vi "GetViableCoordinate.vi"(2 "Target Region [0-3]":i32, 3 "Actual Target Strip [0-1279]":i32) -> (0 "Offset":i32, 1 "Move Probecard to Strip #":i32)   [LabVIEW 2019]
uses:
  ProbePlanParams.vi
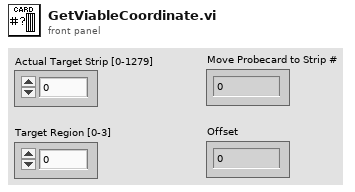
[diagram p1: front panel]
types:
  T1 = cluster{"Strip Number OUT":i32, "X0":i32, "Y0":i32, "X1":i32, "Y1":i32, "Xref":dbl, "Yref":dbl, "ProbePlan type":u32, "Inner pads offset":ext, "Outer pads offset":ext, "l_inner":ext, "l_outer":ext, "strip numbering":u16, "Device Orientation":ext, "Stagger offset":i32, "Yoffset":dbl, "Strip pitch":dbl, "Fiducail separation":dbl, "Radius":ext, "Relative strip angles":dbl, "Probeplan description":string, "ProbePlan array":cluster{"Region":string, "ProbePoints":cluster{"X":dbl, "Y":dbl, "Label":string, "CardViable?":bool}[]}[], "Test ProbePoints":cluster{"Regions Enabled":bool[], "From index":u32[], "To index":u32[]}}
  T2 = cluster{"Region":string, "ProbePoints":cluster{"X":dbl, "Y":dbl, "Label":string, "CardViable?":bool}[]}[]
  T3 = cluster{"Region":string, "ProbePoints":cluster{"X":dbl, "Y":dbl, "Label":string, "CardViable?":bool}[]}
  T4 = cluster{"X":dbl, "Y":dbl, "Label":string, "CardViable?":bool}[]
  T5 = cluster{"X":dbl, "Y":dbl, "Label":string, "CardViable?":bool}
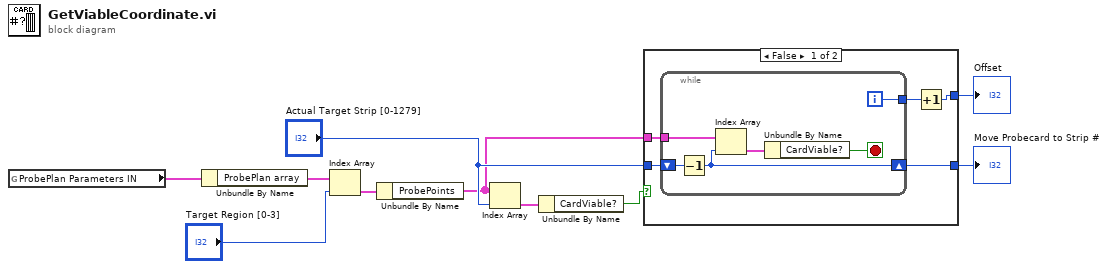
[diagram p0: block diagram]
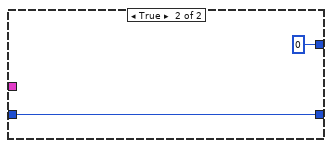
[diagram p2: hidden frame]
diagram:
  n1 = global read "ProbePlanParams.vi" "ProbePlan Parameters IN"() -> (w10:T1)
  n2 = Unbundle By Name(w10) -> ("ProbePlan array"=w9:T2)
  n3 = Index Array(array=w9, index="Target Region [0-3]") -> (element=w7:T3)
  n4 = Unbundle By Name(w7) -> ("ProbePoints"=w2:T4)
  n5 = Index Array(array=w2, index="Actual Target Strip [0-1279]") -> (element=w6:T5)
  n6 = Unbundle By Name(w6) -> ("CardViable?"=w5:bool)
  n7 = case shown="False" w5 {
    tunnel: "Actual Target Strip [0-1279]" -> [w15 w23]
    tunnel: [w13 w23] -> w3
    tunnel: w2 -> [w14 _]
    tunnel: [w12 0] -> w1
    frame False {
      n8 = while {
        tunnel: w14 -> [w21]
        tunnel: [w16] -> w11
        shift-right: [w17] -> w13
        shift-left: w15 -> [w20]
        i -> [w16]
        stop <- w18 stop-if-true
        n9 = Decrement(x=w20) -> (x-1=w17:i32)
        n10 = Index Array(array=w21, index=w17) -> (element=w19:T5)
        n11 = Unbundle By Name(w19) -> ("CardViable?"=w18:bool)
      }
      n12 = Increment(x=w11) -> (x+1=w12:i32)
    }
    frame True {
    }
  }
  "Move Probecard to Strip #" <- w3
  "Offset" <- w1
